vi "Digital Encoder Counter.vi"(9 "DigitalInputDevRef":T1={"DevStatus"={"status"=FALSE, "code"=0, "source"=""}, "DIO Channel"=enum."DIO 1"}, 10 "Previous Count":i32, 11 "Shooter CounterDevRef":T3={"DevStatus"={"status"=FALSE, "code"=0, "source"=""}, "CntIndex"=enum."Invalid"}) -> (1 "DigitalInputDevRef 2":T1={"DevStatus"={"status"=FALSE, "code"=0, "source"=""}, "DIO Channel"=enum."DIO 1"}, 2 "Current Count":i32, 3 "Shooter CounterDevRef 2":T3={"DevStatus"={"status"=FALSE, "code"=0, "source"=""}, "CntIndex"=enum."Invalid"})   [LabVIEW 2015]
uses:
  <vilib>/Rock Robotics/WPI/Counter/WPI_CounterDevRef.ctl
  <vilib>/Rock Robotics/SystemInterfaces/Counter/FPGA_CounterCtrSystemIndex.ctl
  <vilib>/Rock Robotics/WPI/DigitalInput/WPI_DigitalInputDevRef.ctl
  <vilib>/Rock Robotics/SystemInterfaces/DIO/FPGA_DIOChannel.ctl
  <vilib>/Rock Robotics/Network Tables/NT Write Boolean.vi
  Robot Values.vi
  <vilib>/Rock Robotics/Network Tables/NT Write Number.vi
  <vilib>/ptbypt/NI_PtbyPt.lvlib
panel:
  out "x-y 3":dbl
  in  "sample length":i32=25
  in  "PbP":enum16{"Mean", "Median", "None"}(ring)=enum."None"
  out "x-y":dbl
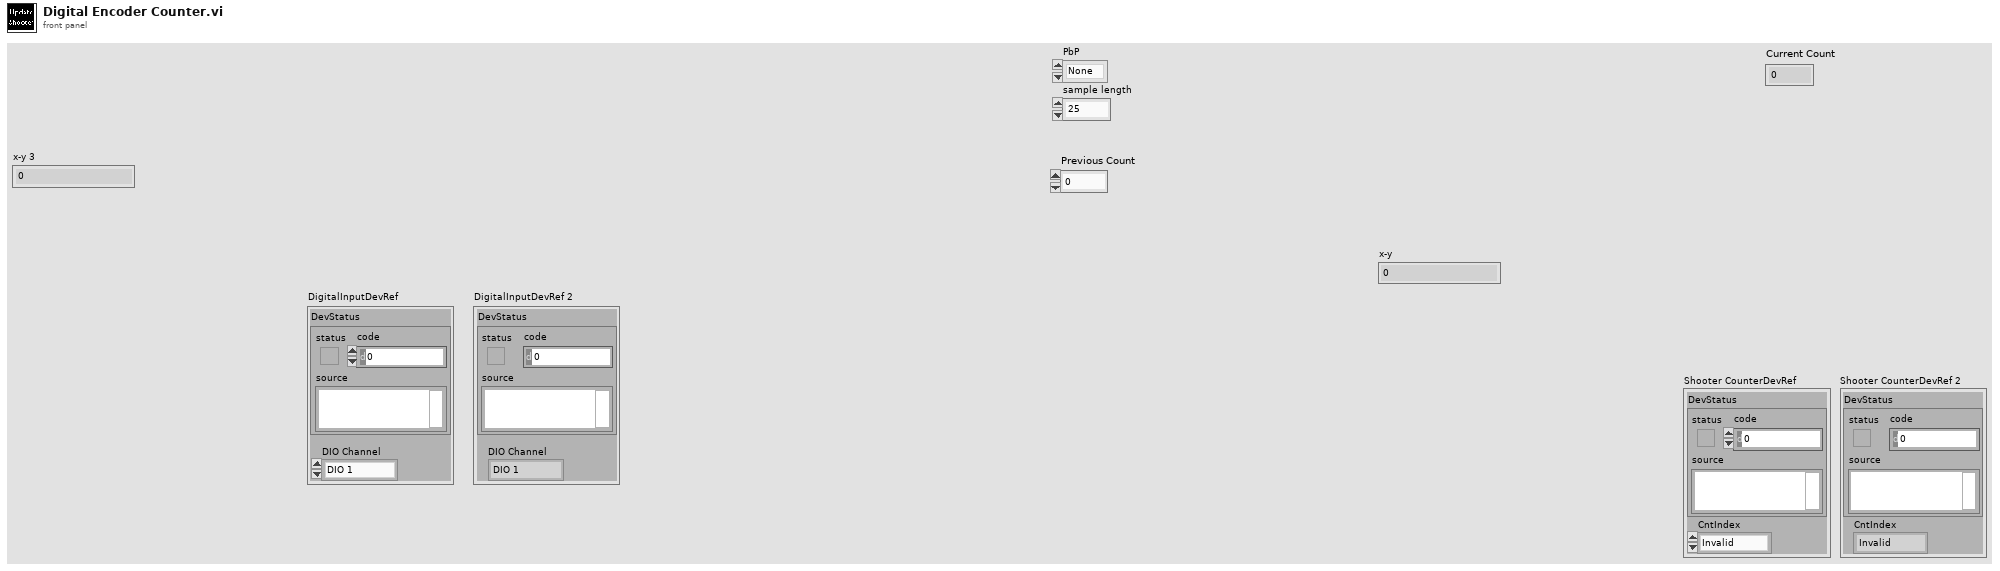
[diagram p1: front panel]
types:
  T1 = typedef "WPI_DigitalInputDevRef.ctl" = cluster{"DevStatus":errorcluster, "DIO Channel":T2}
  T2 = typedef "FPGA_DIOChannel.ctl" = enum8{"DIO 0", "DIO 1", "DIO 2", "DIO 3", "DIO 4", "DIO 5", "DIO 6", "DIO 7", "DIO 8", "DIO 9", "DIO MXP 0", "DIO MXP 1", "DIO MXP 2", "DIO MXP 3", "DIO MXP 4", "DIO MXP 5", "DIO MXP 6", "DIO MXP 7", "DIO MXP 8", "DIO MXP 9", "DIO MXP 10", "DIO MXP 11", "DIO MXP 12", "DIO MXP 13", "DIO MXP 14", "DIO MXP 15", "Invalid"}
  T3 = typedef "WPI_CounterDevRef.ctl" = cluster{"DevStatus":errorcluster, "CntIndex":T4}
  T4 = typedef "FPGA_CounterCtrSystemIndex.ctl" = enum8{"Ctr 0", "Ctr 1", "Ctr 2", "Ctr 3", "Ctr 4", "Ctr 5", "Ctr 6", "Ctr 7", "Invalid"}
  T5 = typedef "Robot Values.ctl" = cluster{"Drive Motors":cluster{"Left Motor Value":dbl, "Right Motor Value":dbl, "Left Motor Encoder":dbl, "Right Motor Encoder":dbl, "High/Low Gear":bool}, "Sensors":cluster{"Gyro Angle":dbl, "Photoeye":bool, "Ultrasonic Range":dbl, "Shooter Speed Encoder":dbl, "Accelerometer Value":dbl, "Flashlight":bool, "Target Distance":dbl, "Target X Value":dbl, "Reset Gyro?":bool}, "Arms":cluster{"Desired Arm Position":dbl, "Left Arm Encoder":dbl, "Right Arm Encoder":dbl, "Left Arm Lower Limit":bool, "Right Arm Lower Limit":bool, "Initialize Arm Position?":bool}, "Acquisition and Scoring":cluster{"Acquiring?":bool, "Current Speed":dbl, "Setpoint Speed":dbl, "Prep Wheels":bool, "Shoot":bool, "Low Eject":bool, "Reverse Shooter Wheel":bool}, "Hanging":cluster{"Pivot Arms":dbl, "PTO":bool, "Left Pivot Encoder":dbl, "Right Pivot Encoder":dbl, "Hanging Pin":bool}}
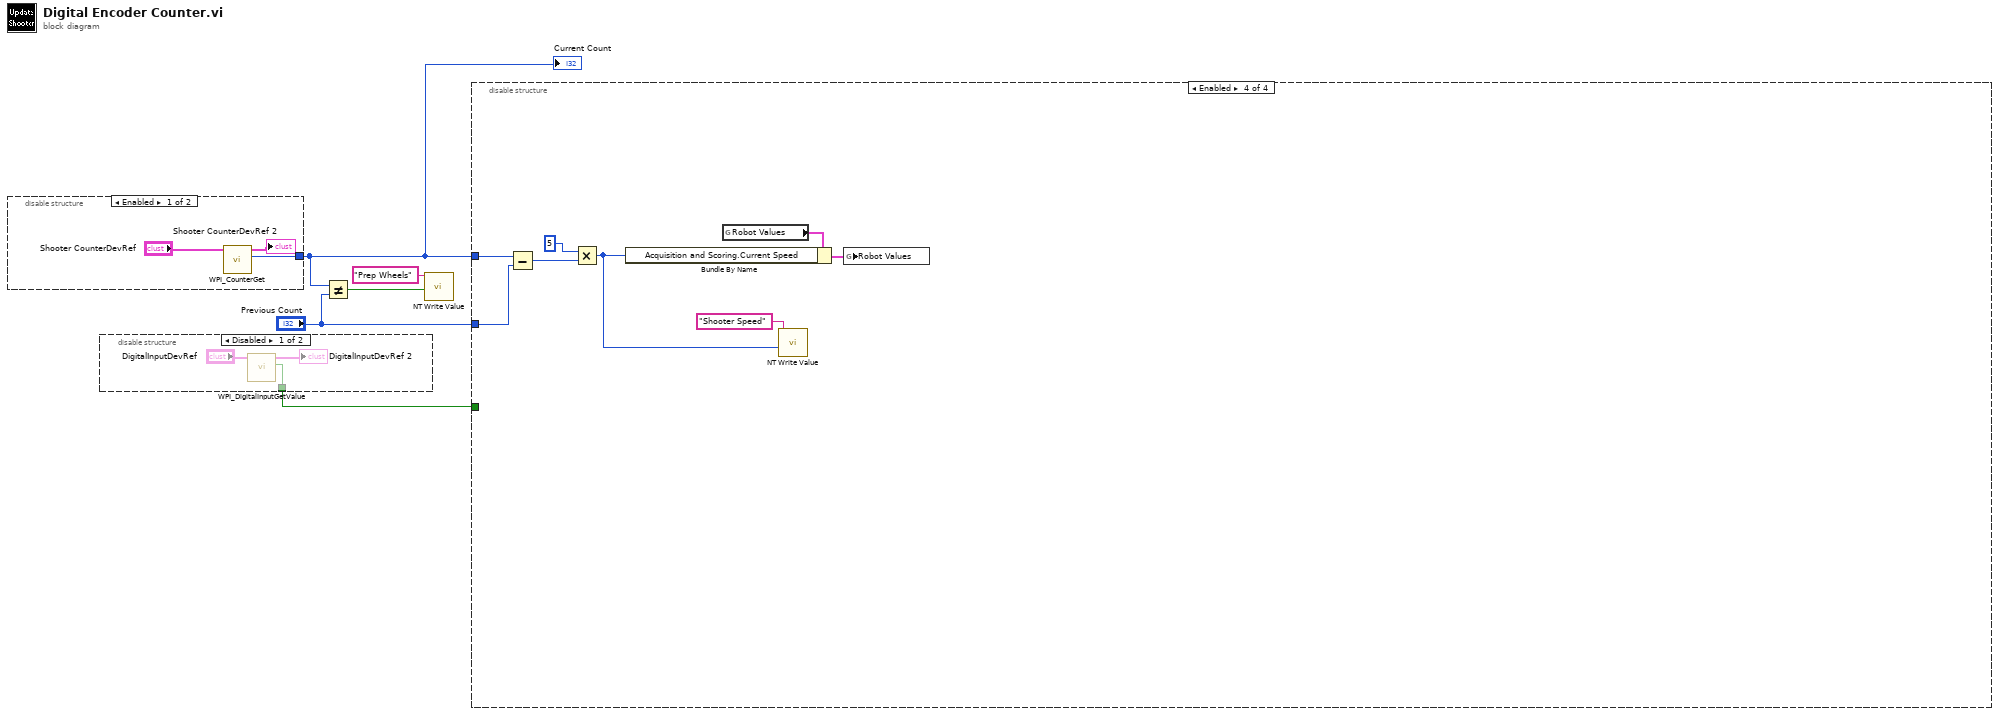
[diagram p0: block diagram]
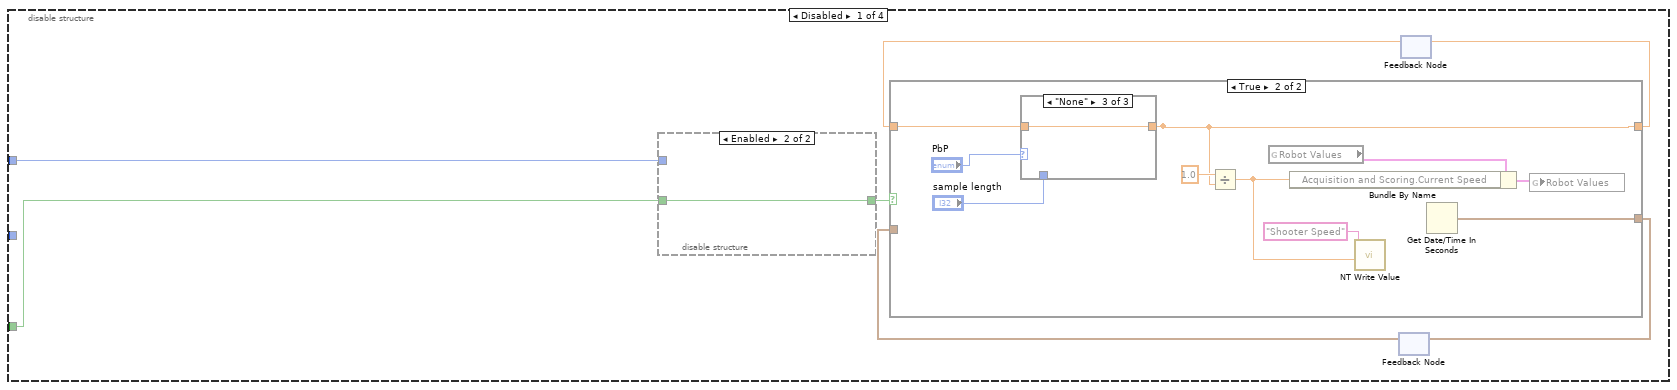
[diagram p4: hidden frame]
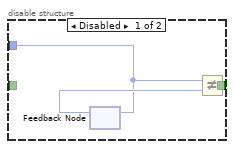
[diagram p5: hidden frame]
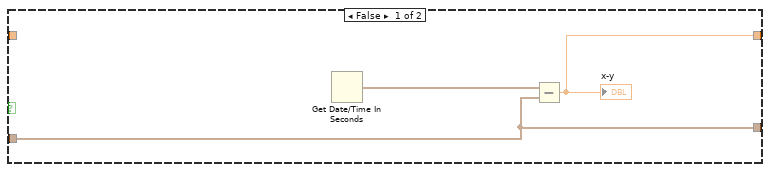
[diagram p6: hidden frame]
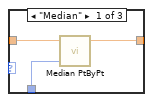
[diagram p7: hidden frame]
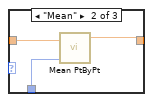
[diagram p8: hidden frame]
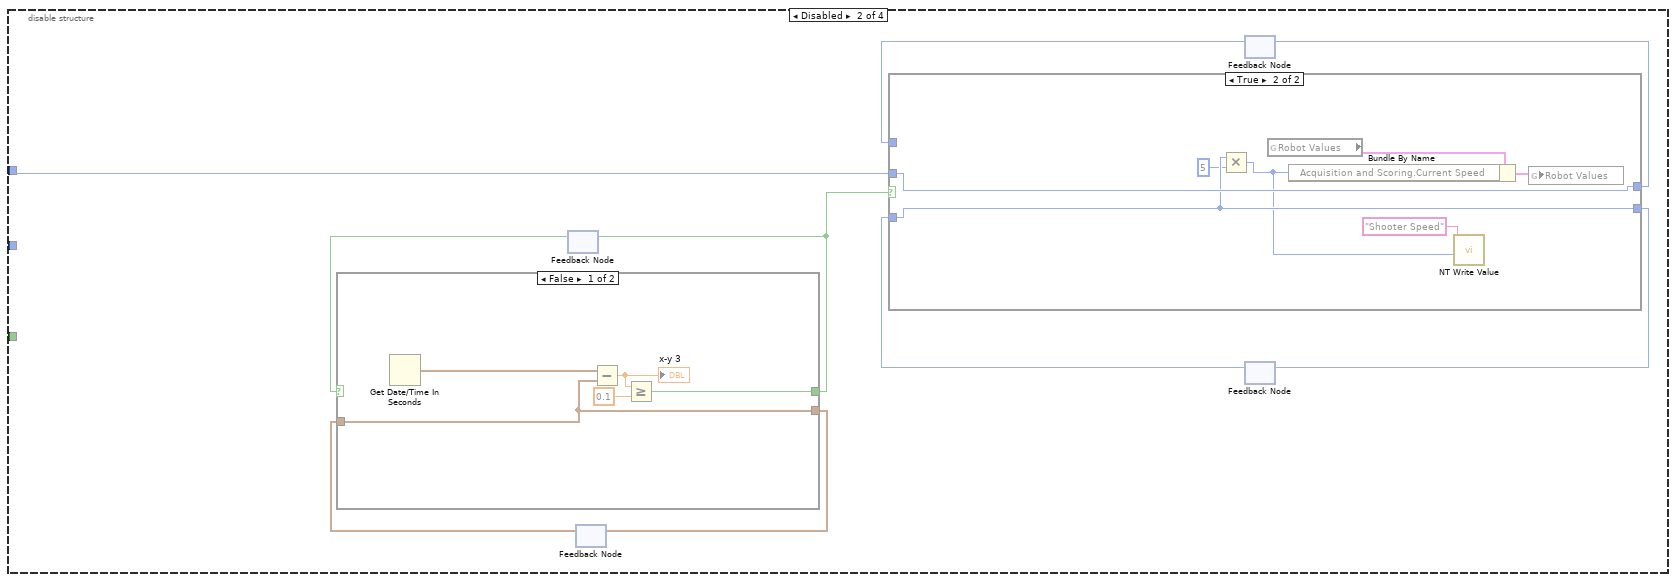
[diagram p9: hidden frame]
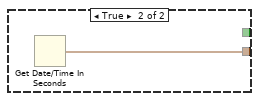
[diagram p10: hidden frame]
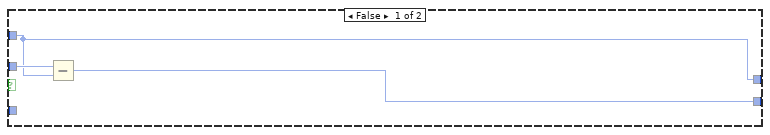
[diagram p11: hidden frame]
diagram:
  n1 = disable-structure shown="Enabled" {
    disable-tunnel: [w6 _] -> w2
    frame Enabled {
      n2 = call <vilib>:"WPI_CounterGet.vi"("CounterDevRef in"="Shooter CounterDevRef") -> ("Value"=w6:i32, "CounterDevRef out"=→"Shooter CounterDevRef 2":T3)  [unwired: 5 in, 4 out]
    }
    frame Disabled {
    }
  }
  "Current Count" <- w2
  n3 = disable-structure shown="Disabled" {
    disable-tunnel: [w9 _] -> w1
    frame Disabled {
      n4 = call <vilib>:"WPI_DigitalInputGetValue.vi"("DigitalInputDevRef"="DigitalInputDevRef") -> ("Value"=w9:bool, "DigitalInputDevRef"=→"DigitalInputDevRef 2":T1)  [unwired: 8 in, 1 out]
    }
    frame Enabled {
    }
  }
  n5 = Not Equal?(x=w2, y="Previous Count") -> (x != y?=w3:bool)
  n6 = call-poly <vilib>:"NT Write Value.vi"("Boolean"=w3, "Name"="Prep Wheels") -> ()  [unwired: 9 in, 1 out]
  n7 = disable-structure shown="Enabled" {
    disable-tunnel: w2 -> [w13 w43 _ w72]
    disable-tunnel: "Previous Count" -> [_ _ _ w70]
    disable-tunnel: w1 -> [w12 _ _ _]
    frame Disabled {
      n8 = disable-structure shown="Enabled" {
        disable-tunnel: [w21 w22] -> w15
        disable-tunnel: w13 -> [w19 _]
        disable-tunnel: w12 -> [_ w22]
        frame Disabled {
          n9 = feedback #1() -> (w20:i32)  [unwired: 1 in]
          n10 = feedback-in #1(w19) -> ()
          n11 = Not Equal?(x=w19, y=w20) -> (x != y?=w21:bool)
        }
        frame Enabled {
        }
      }
      n12 = feedback #2() -> (w17:timestamp)  [unwired: 1 in]
      n13 = feedback #3() -> (w16:dbl)  [unwired: 1 in]
      n14 = case shown="True" w15 {
        tunnel: [w24 w35] -> w18
        tunnel: w17 -> [w24 _]
        tunnel: [w23 w26] -> w14
        tunnel: w16 -> [_ w27]
        frame False {
          n15 = Get Date/Time In Seconds() -> (seconds since 1Jan1904=w25:timestamp)
          n16 = Subtract(x=w25, y=w24) -> (x-y=w23:dbl)
          "x-y" <- w23
        }
        frame True {
          n17 = case shown="\"None\"" "PbP" {
            tunnel: w27 -> [w38 w41 w42]
            tunnel: [w37 w40 w42] -> w26
            tunnel: "sample length" -> [w36 w39 _]
            frame "Median" {
              n18 = call <vilib>:"Median PtByPt.vi"("sample length"=w36, "x"=w38) -> ("median"=w37:dbl)  [unwired: 2 in, 1 out]
            }
            frame "Mean" {
              n19 = call <vilib>:"Mean PtByPt.vi"("x"=w41, "sample length"=w39) -> ("mean"=w40:dbl)  [unwired: 2 in, 1 out]
            }
            frame "None" {
            }
          }
          n20 = Divide(x=1.0, y=w26) -> (x/y=w29:dbl)
          n21 = global read "Robot Values.vi" "Robot Values"() -> (w33:T5)
          n22 = Bundle By Name(cluster=w33, "Acquisition and Scoring.Current Speed"=w29) -> (w32:T5)
          n23 = call-poly <vilib>:"NT Write Value.vi"("Numeric"=w29, "Name"="Shooter Speed") -> ()  [unwired: 9 in, 1 out]
          n24 = Get Date/Time In Seconds() -> (seconds since 1Jan1904=w35:timestamp)
          n25 = global write "Robot Values.vi" "Robot Values"(w32) -> ()
        }
      }
      n26 = feedback-in #2(w18) -> ()
      n27 = feedback-in #3(w14) -> ()
    }
    frame Disabled {
      n28 = feedback #4() -> (w49:bool)  [unwired: 1 in]
      n29 = feedback #5() -> (w50:timestamp)  [unwired: 1 in]
      n30 = case shown="False" w49 {
        tunnel: [w55 w57] -> w51
        tunnel: w50 -> [w55 _]
        tunnel: [w52 _] -> w48
        frame False {
          n31 = Get Date/Time In Seconds() -> (seconds since 1Jan1904=w56:timestamp)
          n32 = Subtract(x=w56, y=w55) -> (x-y=w54:dbl)
          "x-y 3" <- w54
          n33 = Greater Or Equal?(x=w54, y=0.1) -> (x >= y?=w52:bool)
        }
        frame True {
          n34 = Get Date/Time In Seconds() -> (seconds since 1Jan1904=w57:timestamp)
        }
      }
      n35 = feedback-in #4(w48) -> ()
      n36 = feedback-in #5(w51) -> ()
      n37 = feedback #6() -> (w46:i32)  [unwired: 1 in]
      n38 = feedback #7() -> (w44:i32)  [unwired: 1 in]
      n39 = case shown="True" w48 {
        tunnel: [w58 w65] -> w47
        tunnel: w46 -> [w58 _]
        tunnel: w43 -> [w60 w65]
        tunnel: [w59 w64] -> w45
        tunnel: w44 -> [_ w64]
        frame False {
          n40 = Subtract(x=w60, y=w58) -> (x-y=w59:i32)
        }
        frame True {
          n41 = Multiply(x=w64, y=5) -> (x*y=w61:i32)
          n42 = global read "Robot Values.vi" "Robot Values"() -> (w67:T5)
          n43 = Bundle By Name(cluster=w67, "Acquisition and Scoring.Current Speed"=w61) -> (w66:T5)
          n44 = call-poly <vilib>:"NT Write Value.vi"("Numeric"=w61, "Name"="Shooter Speed") -> ()  [unwired: 9 in, 1 out]
          n45 = global write "Robot Values.vi" "Robot Values"(w66) -> ()
        }
      }
      n46 = feedback-in #6(w47) -> ()
      n47 = feedback-in #7(w45) -> ()
    }
    frame Disabled {
    }
    frame Enabled {
      n48 = Subtract(x=w72, y=w70) -> (x-y=w71:i32)
      n49 = Multiply(x=5, y=w71) -> (x*y=w68:i32)
      n50 = global read "Robot Values.vi" "Robot Values"() -> (w75:T5)
      n51 = Bundle By Name(cluster=w75, "Acquisition and Scoring.Current Speed"=w68) -> (w74:T5)
      n52 = call-poly <vilib>:"NT Write Value.vi"("Numeric"=w68, "Name"="Shooter Speed") -> ()  [unwired: 9 in, 1 out]
      n53 = global write "Robot Values.vi" "Robot Values"(w74) -> ()
    }
  }
